vi "cfg separate v2 and v3.vi"(8 "error in":errorcluster, 11 "Engine Configuration In":T4[](array[typedef])) -> (0 "error out":errorcluster, 2 "Log Actions":T1(array[cluster]), 3 "Engine Configuration Out":T3(array[cluster]))   [LabVIEW 2013, in "Standard Engine Configuration.lvclass"]
uses:
  Standard Engine Configuration.lvclass
  Module Specific Configuration.ctl
  Module Decimation.ctl
  Runtime/error responses.ctl
  error options.ctl
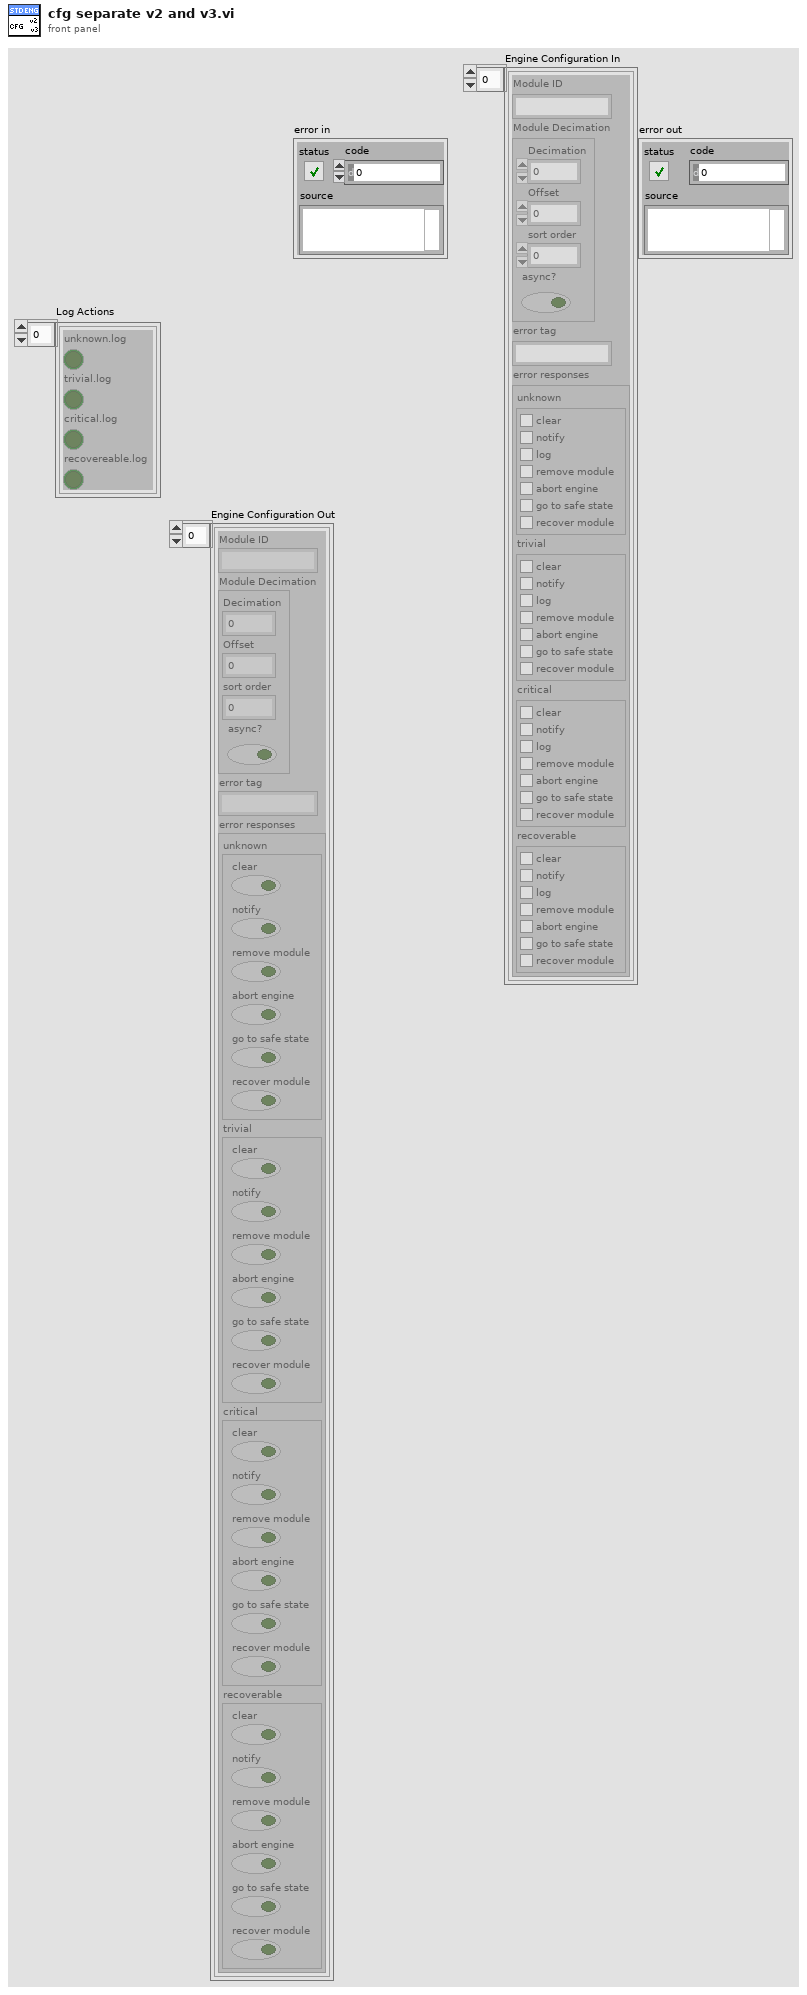
[diagram p1: front panel]
types:
  T1 = cluster{"unknown.log":bool, "trivial.log":bool, "critical.log":bool, "recovereable.log":bool}[]
  T2 = typedef "Standard Engine Configuration.lvclass/Module Decimation.ctl" = cluster{"Decimation":u16, "Offset":u16, "sort order":i32, "async?":bool}
  T3 = cluster{"Module ID":string, "Module Decimation":T2, "error tag":string, "error responses":cluster{"unknown":cluster{"clear":bool, "notify":bool, "remove module":bool, "abort engine":bool, "go to safe state":bool, "recover module":bool}, "trivial":cluster{"clear":bool, "notify":bool, "remove module":bool, "abort engine":bool, "go to safe state":bool, "recover module":bool}, "critical":cluster{"clear":bool, "notify":bool, "remove module":bool, "abort engine":bool, "go to safe state":bool, "recover module":bool}, "recoverable":cluster{"clear":bool, "notify":bool, "remove module":bool, "abort engine":bool, "go to safe state":bool, "recover module":bool}}}[]
  T4 = typedef "Standard Engine Configuration.lvclass/Module Specific Configuration.ctl" = cluster{"Module ID":string, "Module Decimation":T2, "error tag":string, "error responses":T5}
  T5 = typedef "Standard Engine Configuration.lvclass/error responses.ctl" = cluster{"unknown":T6, "trivial":T6, "critical":T6, "recoverable":T6}
  T6 = typedef "Standard Engine Configuration.lvclass/error options.ctl" = cluster{"clear":bool, "notify":bool, "log":bool, "remove module":bool, "abort engine":bool, "go to safe state":bool, "recover module":bool}
  T7 = cluster{"unknown.log":bool, "trivial.log":bool, "critical.log":bool, "recovereable.log":bool}
  T8 = cluster{"Module ID":string, "Module Decimation":T2, "error tag":string, "error responses":cluster{"unknown":cluster{"clear":bool, "notify":bool, "remove module":bool, "abort engine":bool, "go to safe state":bool, "recover module":bool}, "trivial":cluster{"clear":bool, "notify":bool, "remove module":bool, "abort engine":bool, "go to safe state":bool, "recover module":bool}, "critical":cluster{"clear":bool, "notify":bool, "remove module":bool, "abort engine":bool, "go to safe state":bool, "recover module":bool}, "recoverable":cluster{"clear":bool, "notify":bool, "remove module":bool, "abort engine":bool, "go to safe state":bool, "recover module":bool}}}
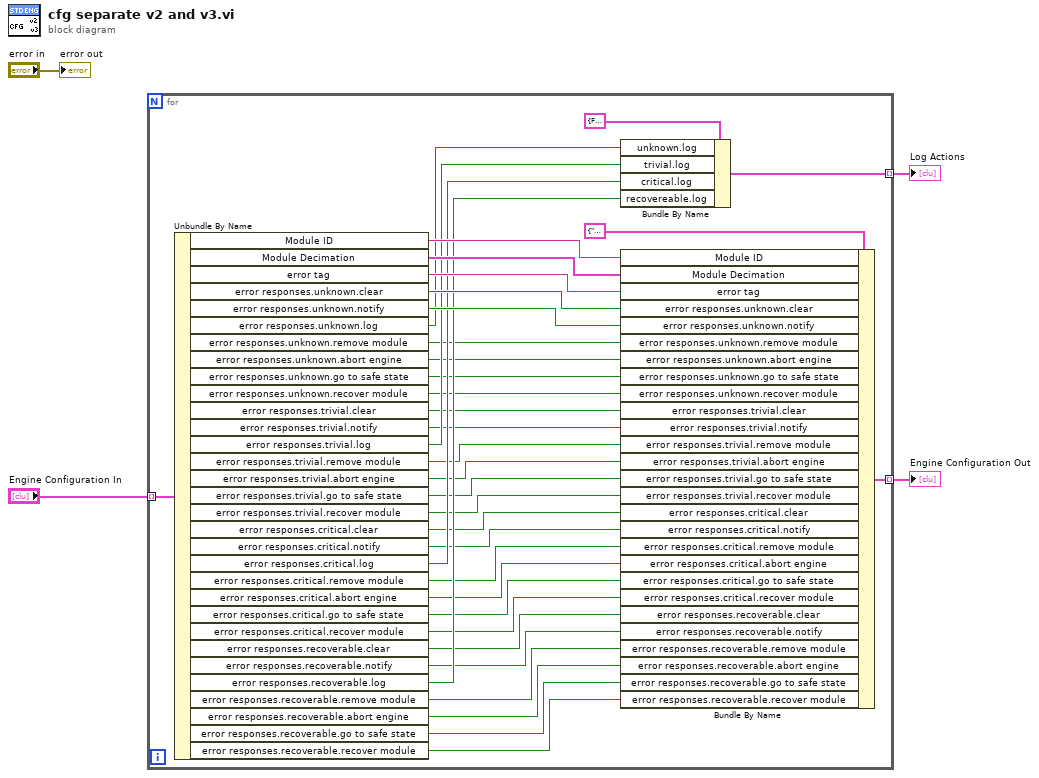
[diagram p0: block diagram]
diagram:
  n1 = for {
    tunnel: "Engine Configuration In" -> [w40] mode=indexing
    tunnel: [w39] -> w3 mode=indexing
    tunnel: [w31] -> w1 mode=indexing
    n2 = Unbundle By Name(w40) -> ("Module ID"=w38:string, "Module Decimation"=w37:T2, "error tag"=w36:string, "error responses.unknown.clear"=w35:bool, "error responses.unknown.notify"=w34:bool, "error responses.unknown.log"=w30:bool, "error responses.unknown.remove module"=w26:bool, "error responses.unknown.abort engine"=w25:bool, "error responses.unknown.go to safe state"=w24:bool, "error responses.unknown.recover module"=w23:bool, "error responses.trivial.clear"=w22:bool, "error responses.trivial.notify"=w21:bool, "error responses.trivial.log"=w29:bool, "error responses.trivial.remove module"=w20:bool, "error responses.trivial.abort engine"=w19:bool, "error responses.trivial.go to safe state"=w18:bool, "error responses.trivial.recover module"=w17:bool, "error responses.critical.clear"=w16:bool, "error responses.critical.notify"=w15:bool, "error responses.critical.log"=w28:bool, "error responses.critical.remove module"=w14:bool, "error responses.critical.abort engine"=w13:bool, "error responses.critical.go to safe state"=w12:bool, "error responses.critical.recover module"=w11:bool, "error responses.recoverable.clear"=w10:bool, "error responses.recoverable.notify"=w9:bool, "error responses.recoverable.log"=w27:bool, "error responses.recoverable.remove module"=w8:bool, "error responses.recoverable.abort engine"=w7:bool, "error responses.recoverable.go to safe state"=w6:bool, "error responses.recoverable.recover module"=w5:bool)
    n3 = Bundle By Name(cluster=T7 {"unknown.log"=FALSE, "trivial.log"=FALSE, "critical.log"=FALSE, "recovereable.log"=FALSE} ("Error Responses"), "unknown.log"=w30, "trivial.log"=w29, "critical.log"=w28, "recovereable.log"=w27) -> (w31:T7)
    n4 = Bundle By Name(cluster=T8 {"Module ID"="", "Module Decimation"={"Decimation"=0, "Offset"=0, "sort order"=0, "async?"=FALSE}, "error tag"="", "error responses"={"unknown"={"clear"=FALSE, "notify"=FALSE, "remove module"=FALSE, "abort engine"=FALSE, "go to safe state"=FALSE, "recover module"=FALSE}, "trivial"={"clear"=FALSE, "notify"=FALSE, "remove module"=FALSE, "abort engine"=FALSE, "go to safe state"=FALSE, "recover module"=FALSE}, "critical"={"clear"=FALSE, "notify"=FALSE, "remove module"=FALSE, "abort engine"=FALSE, "go to safe state"=FALSE, "recover module"=FALSE}, "recoverable"={"clear"=FALSE, "notify"=FALSE, "remove module"=FALSE, "abort engine"=FALSE, "go to safe state"=FALSE, "recover module"=FALSE}}} ("Module Specific Configuration"), "Module ID"=w38, "Module Decimation"=w37, "error tag"=w36, "error responses.unknown.clear"=w35, "error responses.unknown.notify"=w34, "error responses.unknown.remove module"=w26, "error responses.unknown.abort engine"=w25, "error responses.unknown.go to safe state"=w24, "error responses.unknown.recover module"=w23, "error responses.trivial.clear"=w22, "error responses.trivial.notify"=w21, "error responses.trivial.remove module"=w20, "error responses.trivial.abort engine"=w19, "error responses.trivial.go to safe state"=w18, "error responses.trivial.recover module"=w17, "error responses.critical.clear"=w16, "error responses.critical.notify"=w15, "error responses.critical.remove module"=w14, "error responses.critical.abort engine"=w13, "error responses.critical.go to safe state"=w12, "error responses.critical.recover module"=w11, "error responses.recoverable.clear"=w10, "error responses.recoverable.notify"=w9, "error responses.recoverable.remove module"=w8, "error responses.recoverable.abort engine"=w7, "error responses.recoverable.go to safe state"=w6, "error responses.recoverable.recover module"=w5) -> (w39:T8)
  }
  "Engine Configuration Out" <- w3
  "Log Actions" <- w1
  "error out" <- "error in"
